vi "Convert2MDCMD.vi"(11 "New_Write_CMD":T2={"Data"=0.0, "Register"="", "DataType"="", "Address"="", "Protocol"="", "IOAddress"={"Register"=0, "Address"=0, "Device"=0, "Length"=0, "Offset"=0}, "WriteMode"="0"}) -> (3 "MBWriteCMD":T1={"Function Code"=1, "Starting Address"=0, "Quantity"=0, "Data"=[], "Discrete"=[], "Index of Tags"=[]} {"Function Code" items=["Read Coils"=1, "Read Discrete Inputs"=2, "Read Holding Registers"=3, "Read Input Registers"=4, "Write Single Coil"=5, "Write Single Register"=6, "Read Exception Status"=7, "Write Multiple Coils"=15, "Write Multiple Registers"=16]})   [LabVIEW 2020, in "ModBusCommon.lvlib"]
uses:
  ModBusCommon.lvlib
  DynamicIOCMD/DynamicIOCMD.ctl
  DriverCommon/MB Modbus Command.ctl
  DriverCommon.lvlib
  DynamicIOCMD.lvlib
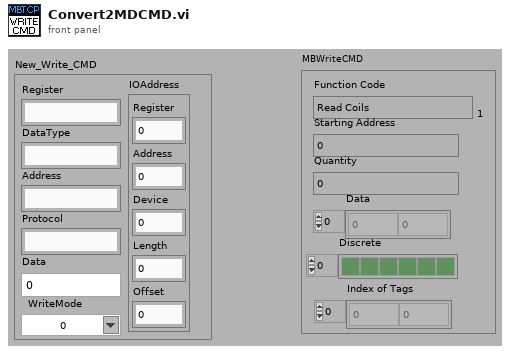
[diagram p1: front panel]
types:
  T1 = typedef "DriverCommon.lvlib/MB Modbus Command.ctl" = cluster{"Function Code":u8, "Starting Address":u16, "Quantity":u16, "Data":u16[], "Discrete":bool[], "Index of Tags":i32[]}
  T2 = typedef "DynamicIOCMD.lvlib/DynamicIOCMD.ctl" = cluster{"Data":dbl, "Register":string, "DataType":string, "Address":string, "Protocol":string, "IOAddress":cluster{"Register":i32, "Address":i32, "Device":i32, "Length":i32, "Offset":i32}, "WriteMode":string}
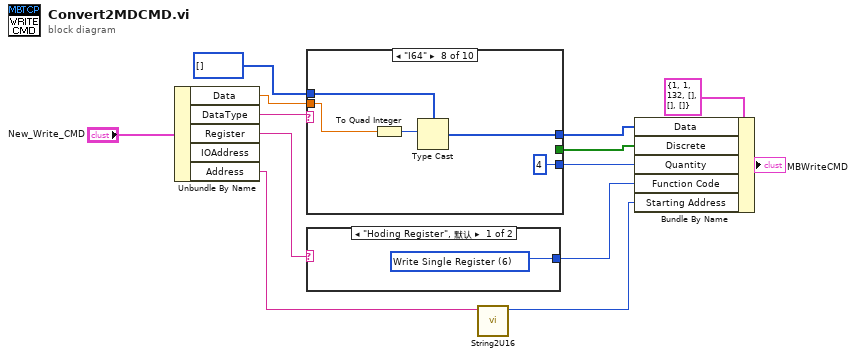
[diagram p0: block diagram]
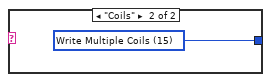
[diagram p2: hidden frame]
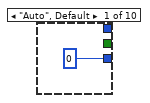
[diagram p3: hidden frame]
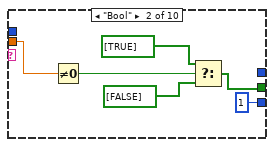
[diagram p4: hidden frame]
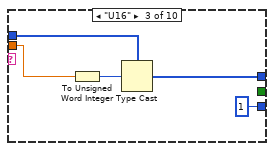
[diagram p5: hidden frame]
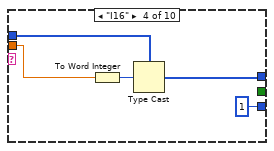
[diagram p6: hidden frame]
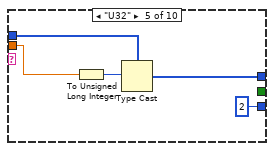
[diagram p7: hidden frame]
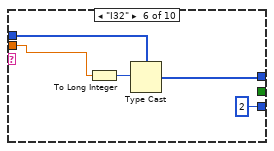
[diagram p8: hidden frame]
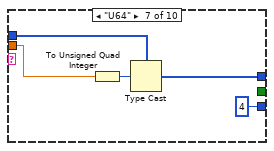
[diagram p9: hidden frame]
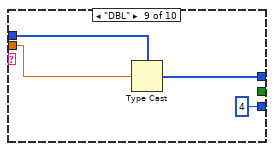
[diagram p10: hidden frame]
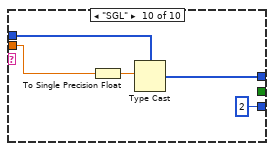
[diagram p11: hidden frame]
diagram:
  n1 = Unbundle By Name("New_Write_CMD") -> ("Data"=w8:dbl, "DataType"=w13:string, "Register"=w9:string, "Address"=w2:string)  [unwired: 1 out]
  n2 = case shown="\"I64\"" w13 {
    tunnel: [_ _ w25 w30 w35 w40 w44 w50 w53 w58] -> w10
    tunnel: u16[] [] ("Value 2") -> [_ _ w24 w29 w34 w39 w45 w49 w54 w59]
    tunnel: w8 -> [_ w18 w22 w27 w32 w37 w42 w47 w52 w56]
    tunnel: [_ w16 _ _ _ _ _ _ _ _] -> w5
    tunnel: [u16 0 ("Quantity") u16 1 ("Quantity") u16 1 ("Quantity") u16 1 ("Quantity") u16 2 ("Quantity") u16 2 ("Quantity") u16 4 ("Quantity") u16 4 ("Quantity") u16 4 ("Quantity") u16 2 ("Quantity")] -> w4
    frame "Auto", Default {
    }
    frame "Bool" {
      n3 = Not Equal To 0?(x=w18) -> (x != 0?=w17:bool)
      n4 = Select(t=bool[] [TRUE] ("Value"), s=w17, f=bool[] [FALSE]) -> (s? t:f=w16:bool[])
    }
    frame "U16" {
      n5 = To Unsigned Word Integer(number=w22) -> (unsigned 16bit integer=w23:u16)
      n6 = Type Cast(type=w24, x=w23) -> (*(type *) &x=w25:u16[])
    }
    frame "I16" {
      n7 = To Word Integer(number=w27) -> (16bit integer=w28:i16)
      n8 = Type Cast(type=w29, x=w28) -> (*(type *) &x=w30:u16[])
    }
    frame "U32" {
      n9 = To Unsigned Long Integer(number=w32) -> (unsigned 32bit integer=w33:u32)
      n10 = Type Cast(type=w34, x=w33) -> (*(type *) &x=w35:u16[])
    }
    frame "I32" {
      n11 = To Long Integer(number=w37) -> (32bit integer=w38:i32)
      n12 = Type Cast(type=w39, x=w38) -> (*(type *) &x=w40:u16[])
    }
    frame "U64" {
      n13 = To Unsigned Quad Integer(1:w42) -> (0:w43:u64)
      n14 = Type Cast(type=w45, x=w43) -> (*(type *) &x=w44:u16[])
    }
    frame "I64" {
      n15 = To Quad Integer(1:w47) -> (0:w48:i64)
      n16 = Type Cast(type=w49, x=w48) -> (*(type *) &x=w50:u16[])
    }
    frame "DBL" {
      n17 = Type Cast(type=w54, x=w52) -> (*(type *) &x=w53:u16[])
    }
    frame "SGL" {
      n18 = To Single Precision Float(number=w56) -> (single precision float=w57:sgl)
      n19 = Type Cast(type=w59, x=w57) -> (*(type *) &x=w58:u16[])
    }
  }
  n20 = case shown="\"Hoding Register\", 默认" w9 {
    tunnel: [w60 w61] -> w6
    frame "Hoding Register", Default {
      w60 = u8 6 items=["Read Coils"=1, "Read Discrete Inputs"=2, "Read Holding Registers"=3, "Read Input Registers"=4, "Write Single Coil"=5, "Write Single Register"=6, "Read Exception Status"=7, "Write Multiple Coils"=15, "Write Multiple Registers"=16] ("Function Code")
    }
    frame "Coils" {
      w61 = u8 15 items=["Read Coils"=1, "Read Discrete Inputs"=2, "Read Holding Registers"=3, "Read Input Registers"=4, "Write Single Coil"=5, "Write Single Register"=6, "Read Exception Status"=7, "Write Multiple Coils"=15, "Write Multiple Registers"=16] ("Function Code")
    }
  }
  n21 = call "String2U16.vi"("String"=w2) -> ("U16"=w1:u16)  [unwired: 10 in]
  n22 = Bundle By Name(cluster=T1 {"Function Code"=1, "Starting Address"=1, "Quantity"=132, "Data"=[], "Discrete"=[], "Index of Tags"=[]} ("New_Write_CMD"), "Data"=w10, "Discrete"=w5, "Quantity"=w4, "Function Code"=w6, "Starting Address"=w1) -> (→"MBWriteCMD":T1)
